vi "Get VPA 1 Values.vi"(0 "Controller #":u16, 1 "Command 1":string="MG DPcur", 2 "Command 2":string="MG MLtot", 3 "SimOn":bool, 5 "Prev Delta-P":dbl format="%.4f", 7 "Prev Volume":dbl format="%.4f", 9 "No Galil":bool, 11 "ErrIn":errorcluster, 12 "Iteration":i32, 13 "Initialize":bool, 14 "Stop":bool) -> (4 "hDmc":u32, 6 "Delta-P":dbl format="%.4f", 8 "Volume":dbl format="%.4f", 15 "ErrOut":errorcluster)   [LabVIEW 2013]
uses:
  DMC32.dll
panel:
  in  "VI Name":string="Get VPA 1 Values.vi"
  out "Command 2 Err":i32
  out "Response 2":string
  out "Close Err":i32
  out "Command 1 Err":i32
  out "Open Err":i32
  out "Response 1":string
  # "Notes:\n1) The five \"Get VPA x values.vi\"\n     are identical except for their\n     name and \"VI Name\" text.\n2) This vi automatically opens and\n    closes a Galil session whenever\n    the \"No Galil\" value changes in\n    the middle of a test."
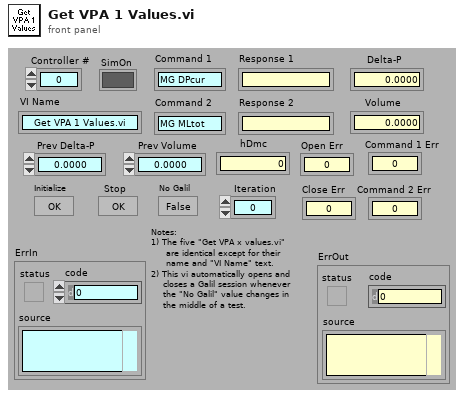
[diagram p1: front panel]
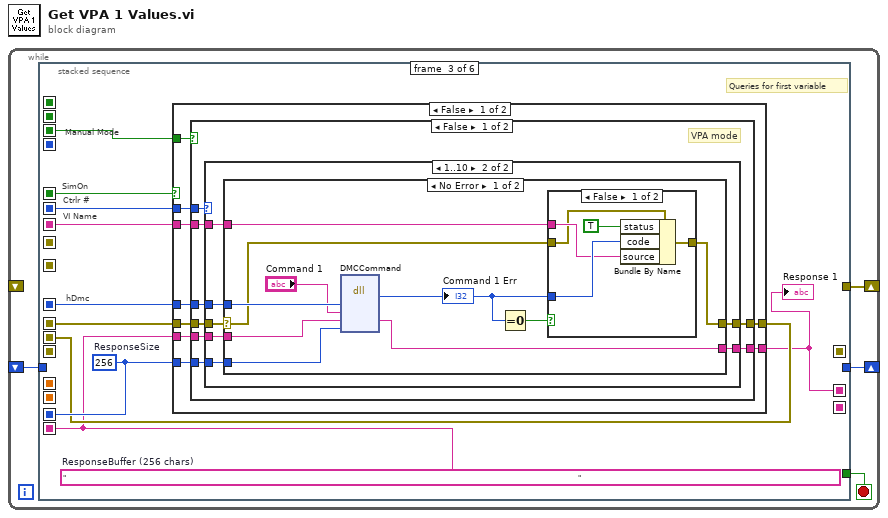
[diagram p0: block diagram]
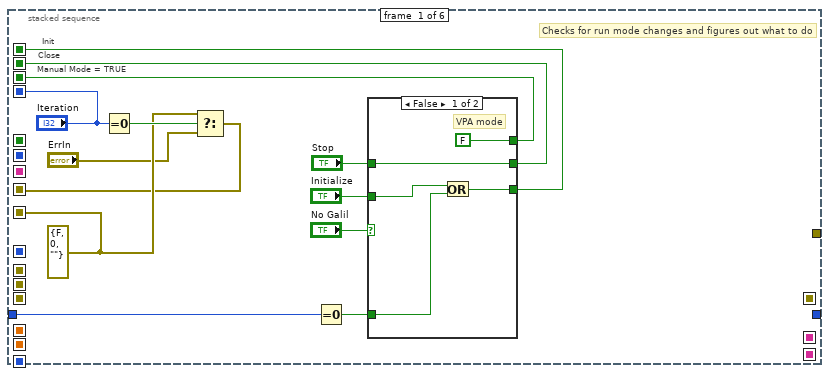
[diagram p2: hidden frame]
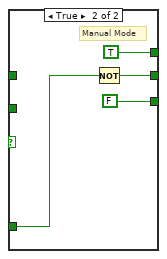
[diagram p3: hidden frame]
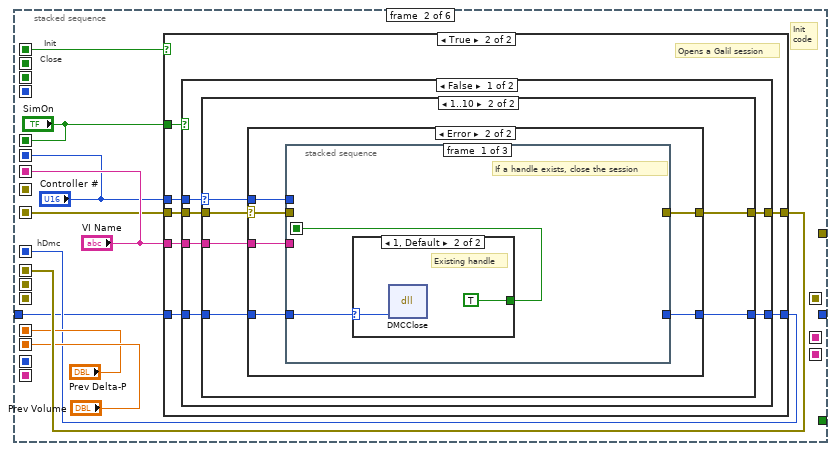
[diagram p4: hidden frame]
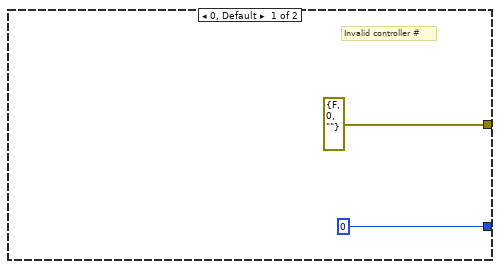
[diagram p6: hidden frame]
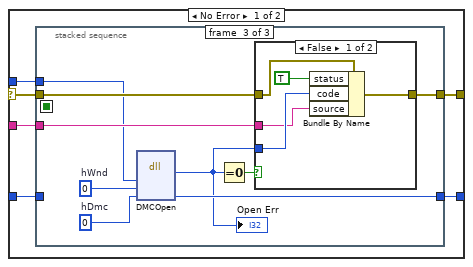
[diagram p7: hidden frame]
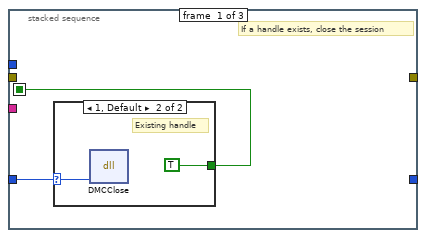
[diagram p8: hidden frame]
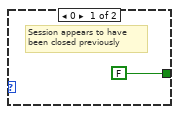
[diagram p9: hidden frame]
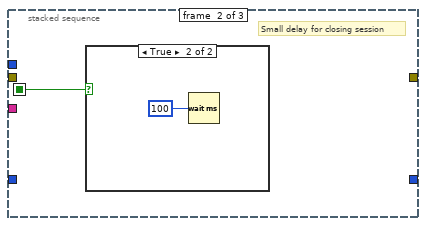
[diagram p10: hidden frame]
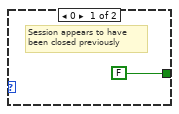
[diagram p13: hidden frame]
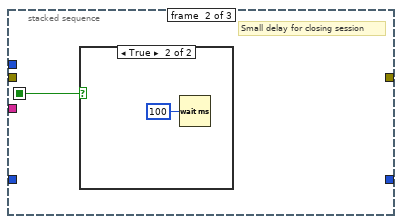
[diagram p14: hidden frame]
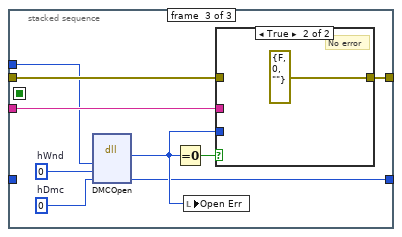
[diagram p16: hidden frame]
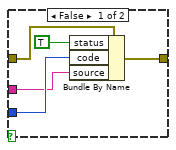
[diagram p17: hidden frame]
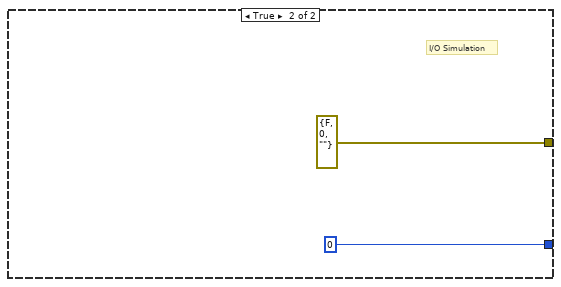
[diagram p18: hidden frame]
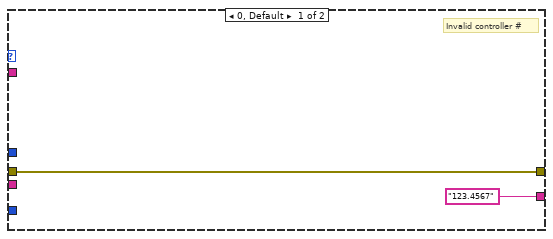
[diagram p19: hidden frame]
diagram:
  n1 = while {
    shift-right: [w4] -> _
    shift-left: _ -> [w3]
    shift-right: [w1] -> _
    shift-left: _ -> [_]
    stop <- w2 stop-if-true
    n2 = stacked-sequence {
      seq-local: [_ w32 _ _ _ _] -> [_ _ w127 w185 w241 w279]
      seq-local: [_ _ w120 _ _ _] -> [_ _ _ w184 _ _]
      seq-local: [_ _ w126 _ _ _] -> [_ _ _ w183 _ _]
      seq-local: [_ w36 _ _ _ _] -> [_ _ w125 _ _ _]
      seq-local: [_ "VI Name" _ _ _ _] -> [_ _ w124 w181 w239 _]
      seq-local: [_ _ w123 _ _ _] -> [_ _ _ w182 _ _]
      seq-local: [_ _ _ w180 _ _] -> [_ _ _ _ w240 _]
      seq-local: [_ "SimOn" _ _ _ _] -> [_ _ w122 w179 w237 _]
      seq-local: [_ _ w121 _ _ _] -> [_ _ _ _ _ w286]
      seq-local: [_ _ _ w178 _ _] -> [_ _ _ _ _ w284]
      seq-local: [_ _ _ _ w238 _] -> [_ _ _ _ _ w276]
      seq-local: [_ "Prev Delta-P" _ _ _ _] -> [_ _ _ _ _ w282]
      seq-local: [_ "Prev Volume" _ _ _ _] -> [_ _ _ _ _ w281]
      seq-local: [_ "Controller #" _ _ _ _] -> [_ _ w119 w177 w236 _]
      seq-local: [w13 _ _ _ _ _] -> [_ w28 _ _ _ _]
      seq-local: [w10 _ _ _ _ _] -> [_ _ _ _ w234 _]
      seq-local: [w12 _ _ _ _ _] -> [_ _ w118 w176 _ _]
      seq-local: [w7 _ _ _ _ _] -> [_ w27 _ _ _ _]
      seq-local: ["Iteration" _ _ _ _ _] -> [_ _ _ _ _ _]
      seq-local: [w5 _ _ _ _ _] -> [_ _ _ _ _ w278]
      tunnel: [_ _ _ _ w235 _] -> w4
      tunnel: w3 -> [w16 w30 _ _ _ _]
      tunnel: [_ _ _ _ _ TRUE] -> w2
      tunnel: [_ _ _ _ _ w276] -> w1
      frame #0 {
        w7 = errorcluster {"status"=FALSE, "code"=0, "source"=""} ("ErrIn")
        # "Manual Mode = TRUE"
        # "Close"
        # "Init"
        # "Checks for run mode changes and figures out what to do"
        n3 = Equal To 0?(x="Iteration") -> (x = 0?=w8:bool)
        n4 = Select(t=w7, s=w8, f="ErrIn") -> (s? t:f=w5:errorcluster)
        n5 = Equal To 0?(x=w16) -> (x = 0?=w14:bool)
        n6 = case shown="False" "No Galil" {
          tunnel: "Initialize" -> [w22 _]
          tunnel: w14 -> [w21 w25]
          tunnel: [w20 FALSE] -> w13
          tunnel: [FALSE TRUE] -> w12
          tunnel: "Stop" -> [w19 _]
          tunnel: [w19 w24] -> w10
          frame False {
            # "VPA mode"
            n7 = Or(x=w22, y=w21) -> (x .or. y?=w20:bool)
          }
          frame True {
            # "Manual Mode"
            n8 = Not(x=w25) -> (.not. x?=w24:bool)
          }
        }
      }
      frame #1 {
        # "Close"
        # "Init"
        # "Init\ncode"
        # "hDmc"
        n9 = case shown="True" w28 {
          tunnel: w27 -> [w38 w45]
          tunnel: [w37 w44] -> w32
          tunnel: [w38 w43] -> w36
          tunnel: "VI Name" -> [_ w42]
          tunnel: "SimOn" -> [_ w41]
          tunnel: w30 -> [w37 w39]
          tunnel: "Controller #" -> [_ w40]
          frame False {
          }
          frame True {
            # "Opens a Galil session"
            n10 = case shown="False" w41 {
              tunnel: w45 -> [w51 _]
              tunnel: [w50 u32 0 ("hDmc")] -> w44
              tunnel: [w49 errorcluster {"status"=FALSE, "code"=0, "source"=""} ("ErrIn")] -> w43
              tunnel: w42 -> [w48 _]
              tunnel: w40 -> [w47 _]
              tunnel: w39 -> [w46 _]
              frame False {
                n11 = case shown="1..10" w47 {
                  selector: w47 -> [_ w55]
                  tunnel: w51 -> [_ w59]
                  tunnel: [u32 0 ("hDmc") w58] -> w50
                  tunnel: [errorcluster {"status"=FALSE, "code"=0, "source"=""} ("error IO") w57] -> w49
                  tunnel: w48 -> [_ w56]
                  tunnel: w46 -> [_ w54]
                  frame 0, Default {
                    # "Invalid controller #"
                  }
                  frame 1..10 {
                    n12 = case shown="Error" w59 {
                      selector: w59 -> [w64 w92]
                      tunnel: [w65 w88] -> w58
                      tunnel: [w63 w89] -> w57
                      tunnel: w56 -> [w62 w91]
                      tunnel: w55 -> [w61 w90]
                      tunnel: w54 -> [w60 w93]
                      frame No Error {
                        n13 = stacked-sequence {
                          seq-local: [w66 _ _] -> [_ w71 _]
                          tunnel: [_ _ w79] -> w65
                          tunnel: w64 -> [_ _ w77]
                          tunnel: [_ _ w76] -> w63
                          tunnel: w62 -> [_ _ w74]
                          tunnel: w61 -> [_ _ w73]
                          tunnel: w60 -> [w67 _ _]
                          frame #0 {
                            # "If a handle exists, close the session"
                            n14 = case shown="1, Default" w67 {
                              selector: w67 -> [_ w70]
                              tunnel: [FALSE TRUE] -> w66
                              frame 0 {
                                # "Session appears to have\nbeen closed previously"
                              }
                              frame 1, Default {
                                # "Existing handle"
                                n15 = dll-call lib="C:/Documents and Settings/Steven/My Documents/GitHub/ER/DMC32.DLL" fn="DMCClose"("hDMC"=w70) -> ()  [unwired: 5 in, 2 out]
                              }
                            }
                          }
                          frame #1 {
                            # "Small delay for closing session"
                            n16 = case shown="True" w71 {
                              frame False {
                              }
                              frame True {
                                n17 = Wait (ms)(milliseconds to wait=u32 100) -> ()  [unwired: 1 out]
                              }
                            }
                          }
                          frame #2 {
                            w80 = u32 0  # hDmc
                            w81 = u32 0  # hWnd
                            n18 = dll-call lib="C:/Documents and Settings/Steven/My Documents/GitHub/ER/DMC32.DLL" fn="DMCOpen"("Controller"=w73, "hWnd"=w81, "hDmc"=w80) -> (w75:i32, "hDmc"=w79:u32)  [unwired: 5 in, 2 out]
                            "Open Err" <- w75
                            n19 = Equal To 0?(x=w75) -> (x = 0?=w78:bool)
                            n20 = case shown="False" w78 {
                              tunnel: w77 -> [w86 w87]
                              tunnel: [w85 w87] -> w76
                              tunnel: w75 -> [w83 _]
                              tunnel: w74 -> [w82 _]
                              frame False {
                                n21 = Bundle By Name(cluster=w86, "status"=TRUE, "code"=w83, "source"=w82) -> (w85:errorcluster)
                              }
                              frame True {
                                # "No error"
                              }
                            }
                          }
                        }
                      }
                      frame Error {
                        n22 = stacked-sequence {
                          seq-local: [w94 _ _] -> [_ w99 _]
                          tunnel: w93 -> [w95 _ _]
                          tunnel: w92 -> [_ _ w106]
                          tunnel: w91 -> [_ _ w105]
                          tunnel: w90 -> [_ _ w104]
                          tunnel: [_ _ w103] -> w89
                          tunnel: [_ _ w101] -> w88
                          frame #0 {
                            # "If a handle exists, close the session"
                            n23 = case shown="1, Default" w95 {
                              selector: w95 -> [_ w98]
                              tunnel: [FALSE TRUE] -> w94
                              frame 0 {
                                # "Session appears to have\nbeen closed previously"
                              }
                              frame 1, Default {
                                # "Existing handle"
                                n24 = dll-call lib="C:/Documents and Settings/Steven/My Documents/GitHub/ER/DMC32.DLL" fn="DMCClose"("hDMC"=w98) -> ()  [unwired: 5 in, 2 out]
                              }
                            }
                          }
                          frame #1 {
                            # "Small delay for closing session"
                            n25 = case shown="True" w99 {
                              frame False {
                              }
                              frame True {
                                n26 = Wait (ms)(milliseconds to wait=u32 100) -> ()  [unwired: 1 out]
                              }
                            }
                          }
                          frame #2 {
                            w108 = u32 0  # hDmc
                            w109 = u32 0  # hWnd
                            n27 = dll-call lib="C:/Documents and Settings/Steven/My Documents/GitHub/ER/DMC32.DLL" fn="DMCOpen"("Controller"=w104, "hWnd"=w109, "hDmc"=w108) -> (w102:i32, "hDmc"=w101:u32)  [unwired: 5 in, 2 out]
                            n28 = Equal To 0?(x=w102) -> (x = 0?=w107:bool)
                            n29 = local write "Open Err"(w102) -> ()
                            n30 = case shown="True" w107 {
                              tunnel: w106 -> [w114 _]
                              tunnel: [w113 errorcluster {"status"=FALSE, "code"=0, "source"=""} ("error IO")] -> w103
                              tunnel: w102 -> [w111 _]
                              tunnel: w105 -> [w110 _]
                              frame False {
                                n31 = Bundle By Name(cluster=w114, "status"=TRUE, "code"=w111, "source"=w110) -> (w113:errorcluster)
                              }
                              frame True {
                                # "No error"
                              }
                            }
                          }
                        }
                      }
                    }
                  }
                }
              }
              frame True {
                # "I/O Simulation"
              }
            }
          }
        }
      }
      frame #2 {
        w126 = u32 256  # ResponseSize
        w120 = "                                                                                                                                                                                                                                                                "  # ResponseBuffer (256 chars)
        # "Manual Mode"
        # "SimOn"
        # "Ctrlr #"
        # "VI Name"
        # "Queries for first variable"
        # "hDmc"
        n32 = case shown="False" w122 {
          tunnel: w127 -> [w136 _]
          tunnel: w120 -> [w135 _]
          tunnel: w126 -> [w134 _]
          tunnel: w125 -> [w133 w175]
          tunnel: w124 -> [w132 _]
          tunnel: [w131 w175] -> w123
          tunnel: [w130 "123.4567" ("Response")] -> w121
          tunnel: w119 -> [w129 _]
          tunnel: w118 -> [w128 _]
          frame False {
            n33 = case shown="False" w128 {
              tunnel: w136 -> [w144 _]
              tunnel: w135 -> [w143 _]
              tunnel: w134 -> [w142 _]
              tunnel: w133 -> [w141 w173]
              tunnel: w132 -> [w140 _]
              tunnel: [w139 w173] -> w131
              tunnel: [w138 "0"] -> w130
              tunnel: w129 -> [w137 _]
              frame False {
                # "VPA mode"
                n34 = case shown="1..10" w137 {
                  tunnel: w144 -> [_ w153]
                  tunnel: w143 -> [_ w152]
                  tunnel: w142 -> [_ w151]
                  tunnel: w141 -> [w146 w150]
                  tunnel: w140 -> [_ w149]
                  tunnel: [w146 w148] -> w139
                  tunnel: ["123.4567" ("Response") w147] -> w138
                  frame 0, Default {
                    # "Invalid controller #"
                  }
                  frame 1..10 {
                    n35 = case shown="No Error" w150 {
                      selector: w150 -> [w159 w171]
                      tunnel: w153 -> [w163 _]
                      tunnel: w152 -> [w161 _]
                      tunnel: w151 -> [w160 _]
                      tunnel: [w155 w171] -> w148
                      tunnel: w149 -> [w158 _]
                      tunnel: [w154 "Prev Error" ("Response")] -> w147
                      frame No Error {
                        n36 = dll-call lib="C:/Documents and Settings/Steven/My Documents/GitHub/ER/DMC32.DLL" fn="DMCCommand"("hDmc"=w163, "Command"="Command 1", "Response"=w161, "ResponseSize"=w160) -> (w156:i32, "Response"=w154:string)  [unwired: 6 in, 2 out]
                        "Command 1 Err" <- w156
                        n37 = Equal To 0?(x=w156) -> (x = 0?=w157:bool)
                        n38 = case shown="False" w157 {
                          tunnel: w159 -> [w164 w169]
                          tunnel: [w168 w169] -> w155
                          tunnel: w156 -> [w166 _]
                          tunnel: w158 -> [w165 _]
                          frame False {
                            n39 = Bundle By Name(cluster=w164, "status"=TRUE, "code"=w166, "source"=w165) -> (w168:errorcluster)
                          }
                          frame True {
                            # "No error"
                          }
                        }
                      }
                      frame Error {
                        # "Prev Error"
                      }
                    }
                  }
                }
              }
              frame True {
                # "Manual Mode"
              }
            }
          }
          frame True {
            # "I/O Simulation"
          }
        }
        "Response 1" <- w121
      }
      frame #3 {
        # "Manual Mode"
        # "Ctrlr #"
        # "VI Name"
        # "Queries for second variable"
        # "hDmc"
        n40 = case shown="False" w179 {
          tunnel: w185 -> [w194 _]
          tunnel: w184 -> [w193 _]
          tunnel: w183 -> [w192 _]
          tunnel: w182 -> [w191 w233]
          tunnel: w181 -> [w190 _]
          tunnel: [w189 w233] -> w180
          tunnel: [w188 "65.4321" ("Response")] -> w178
          tunnel: w177 -> [w187 _]
          tunnel: w176 -> [w186 _]
          frame False {
            n41 = case shown="False" w186 {
              tunnel: w194 -> [w202 _]
              tunnel: w193 -> [w201 _]
              tunnel: w192 -> [w200 _]
              tunnel: w191 -> [w199 w231]
              tunnel: w190 -> [w198 _]
              tunnel: [w197 w231] -> w189
              tunnel: [w196 "0"] -> w188
              tunnel: w187 -> [w195 _]
              frame False {
                # "VPA mode"
                n42 = case shown="1..10" w195 {
                  tunnel: w202 -> [_ w211]
                  tunnel: w201 -> [_ w210]
                  tunnel: w200 -> [_ w209]
                  tunnel: w199 -> [w204 w208]
                  tunnel: w198 -> [_ w207]
                  tunnel: [w204 w206] -> w197
                  tunnel: ["65.4321" ("Response") w205] -> w196
                  frame 0, Default {
                    # "Invalid controller #"
                  }
                  frame 1..10 {
                    n43 = case shown="No Error" w208 {
                      selector: w208 -> [w214 w229]
                      tunnel: w211 -> [w221 _]
                      tunnel: w210 -> [w219 _]
                      tunnel: w209 -> [w218 _]
                      tunnel: w207 -> [w217 _]
                      tunnel: [w213 w229] -> w206
                      tunnel: [w212 "Prev Error" ("Response")] -> w205
                      frame No Error {
                        n44 = dll-call lib="C:/Documents and Settings/Steven/My Documents/GitHub/ER/DMC32.DLL" fn="DMCCommand"("hDmc"=w221, "Command"="Command 2", "Response"=w219, "ResponseSize"=w218) -> (w216:i32, "Response"=w212:string)  [unwired: 6 in, 2 out]
                        "Command 2 Err" <- w216
                        n45 = Equal To 0?(x=w216) -> (x = 0?=w215:bool)
                        n46 = case shown="True" w215 {
                          tunnel: w214 -> [w222 w227]
                          tunnel: [w226 w227] -> w213
                          tunnel: w216 -> [w224 _]
                          tunnel: w217 -> [w223 _]
                          frame False {
                            n47 = Bundle By Name(cluster=w222, "status"=TRUE, "code"=w224, "source"=w223) -> (w226:errorcluster)
                          }
                          frame True {
                            # "No error"
                          }
                        }
                      }
                      frame Error {
                        # "Prev Error"
                      }
                    }
                  }
                }
              }
              frame True {
                # "Manual mode"
              }
            }
          }
          frame True {
            # "I/O Simulation"
          }
        }
        "Response 2" <- w178
      }
      frame #4 {
        # "Close"
        # "Ctrlr #"
        # "VI Name"
        # "Closes session as req'd"
        # "hDmc"
        n48 = case shown="True" w234 {
          tunnel: w241 -> [w242 w250]
          tunnel: w240 -> [w243 w249]
          tunnel: w239 -> [_ w248]
          tunnel: [w243 w247] -> w238
          tunnel: w237 -> [_ w246]
          tunnel: w236 -> [_ w245]
          tunnel: [w242 u32 0] -> w235
          frame False {
          }
          frame True {
            n49 = case shown="False" w246 {
              tunnel: w250 -> [w255 _]
              tunnel: w249 -> [w254 w275]
              tunnel: w248 -> [w253 _]
              tunnel: [w252 w275] -> w247
              tunnel: w245 -> [w251 _]
              frame False {
                n50 = case shown="1..10" w251 {
                  tunnel: w255 -> [_ w260]
                  tunnel: w254 -> [w256 w259]
                  tunnel: w253 -> [_ w258]
                  tunnel: [w256 w257] -> w252
                  frame 0, Default {
                    # "Invalid controller #"
                  }
                  frame 1..10 {
                    n51 = case shown="No Error" w259 {
                      selector: w259 -> [w262 w274]
                      tunnel: w260 -> [w266 w273]
                      tunnel: [w261 w274] -> w257
                      tunnel: w258 -> [w265 _]
                      frame No Error {
                        n52 = dll-call lib="C:/Documents and Settings/Steven/My Documents/GitHub/ER/DMC32.DLL" fn="DMCClose"("hDMC"=w266) -> (w264:i32)  [unwired: 4 in, 2 out]
                        "Close Err" <- w264
                        n53 = Equal To 0?(x=w264) -> (x = 0?=w263:bool)
                        n54 = case shown="False" w263 {
                          tunnel: w262 -> [w267 w272]
                          tunnel: [w271 w272] -> w261
                          tunnel: w264 -> [w269 _]
                          tunnel: w265 -> [w268 _]
                          frame False {
                            n55 = Bundle By Name(cluster=w267, "status"=TRUE, "code"=w269, "source"=w268) -> (w271:errorcluster)
                          }
                          frame True {
                            # "No error"
                          }
                        }
                      }
                      frame Error {
                        # "Prev error - try to close session"
                        n56 = dll-call lib="C:/Documents and Settings/Steven/My Documents/GitHub/ER/DMC32.DLL" fn="DMCClose"("hDMC"=w273) -> ()  [unwired: 5 in, 2 out]
                      }
                    }
                  }
                }
              }
              frame True {
                # "I/O Simulation"
              }
            }
          }
        }
      }
      frame #5 {
        # "This vi's current error"
        # "Initial input error"
        # "Final values"
        n57 = case shown="No Error" w276 {
          tunnel: w286 -> [w292 _]
          tunnel: [w291 w293] -> w285
          tunnel: w284 -> [w290 _]
          tunnel: [w289 w293] -> w283
          tunnel: w282 -> [_ _]
          tunnel: w281 -> [_ _]
          frame No Error {
            n58 = Fract/Exp String To Number(string=w290) -> (number=w289:dbl)  [unwired: 3 in, 1 out]
            n59 = Fract/Exp String To Number(string=w292) -> (number=w291:dbl)  [unwired: 3 in, 1 out]
          }
          frame Error {
            w293 = nan
          }
        }
        "Volume" <- w283
        "Delta-P" <- w285
        n60 = case shown="No Error" w278 {
          selector: w278 -> [_ w288]
          tunnel: w276 -> [w287 _]
          tunnel: [w287 w288] -> w277
          frame No Error {
          }
          frame Error {
            # "Returns initial error if there was one"
          }
        }
        "ErrOut" <- w277
        "hDmc" <- w279
      }
    }
  }
